vi "PID-testing.vi"() -> ()   [LabVIEW 2011]
uses:
  <vilib>/addons/control/pid/pid.llb/PID (DBL).vi
  <vilib>/Analysis/coordinate.llb/2D Cartesian Coordinate Rotation (Scalar).vi
  <vilib>/Analysis/NI_AALPro.lvlib
  <vilib>/addons/control/pid/NI_PID_pid.lvlib
panel:
  out "Y speed":dbl
  out "X speed":dbl
  in  "Y rate":dbl
  in  "X rate":dbl
  in  "stop":bool
  in  "Y 3":dbl
  in  "X 3":dbl
  in  "Y 2":dbl
  in  "X 2":dbl
  in  "Speed":dbl
  in  "Ramp":dbl
  in  "Y":dbl
  in  "X":dbl
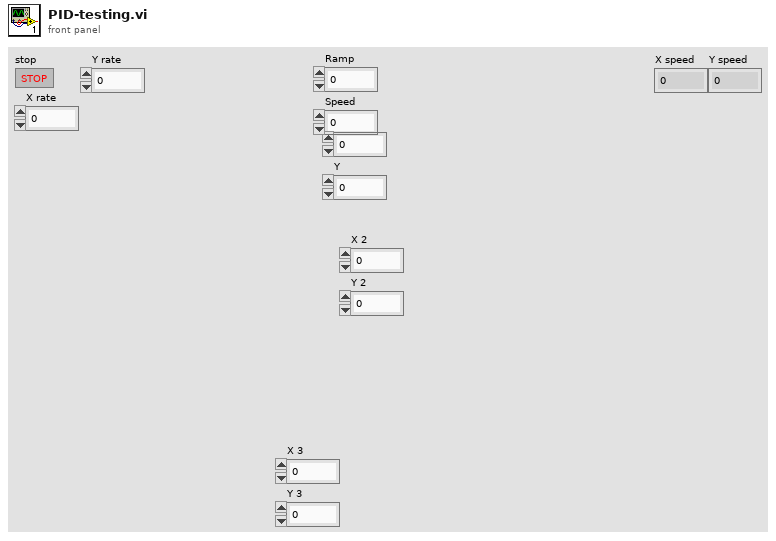
[diagram p1: front panel]
types:
  T1 = cluster{"proportional gain (Kc)":dbl, "integral time (Ti, min)":dbl, "derivative time (Td, min)":dbl}
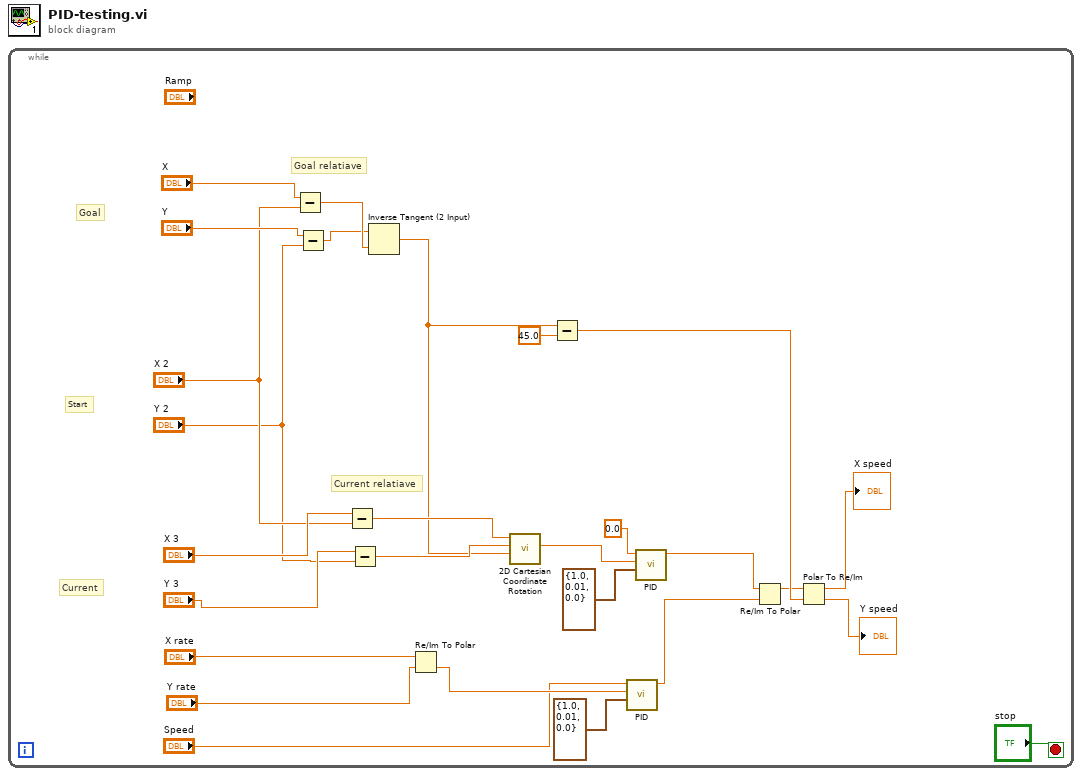
[diagram p0: block diagram]
diagram:
  n1 = while {
    stop <- "stop" stop-if-true
    # "Current relatiave"
    # "Goal relatiave"
    # "Current"
    # "Start"
    # "Goal"
    n2 = Subtract(x="X", y="X 2") -> (x-y=w21:dbl)
    n3 = Subtract(x="Y", y="Y 2") -> (x-y=w20:dbl)
    n4 = Subtract(x="X 3", y="X 2") -> (x-y=w19:dbl)
    n5 = Subtract(x="Y 3", y="Y 2") -> (x-y=w18:dbl)
    n6 = Inverse Tangent (2 Input)(1:w21, 2:w20) -> (0:w12:dbl)
    n7 = Re/Im To Polar(2:"Y rate", 3:"X rate") -> (0:w4:dbl)  [unwired: 1 out]
    n8 = call-poly <vilib>:"2D Cartesian Coordinate Rotation.vi"("theta"=w12, "y"=w18, "x"=w19) -> ("y out"=w8:dbl)  [unwired: 6 in, 2 out]
    n9 = Subtract(x=w12, y=45.0) -> (x-y=w13:dbl)
    n10 = call-poly <vilib>:"PID.vi"("PID gains"=T1 {"proportional gain (Kc)"=1.0, "integral time (Ti, min)"=0.01, "derivative time (Td, min)"=0.0}, "process variable"=w4, "setpoint"="Speed") -> ("output"=w5:dbl)  [unwired: 7 in, 1 out]
    n11 = call-poly <vilib>:"PID.vi"("PID gains"=T1 {"proportional gain (Kc)"=1.0, "integral time (Ti, min)"=0.01, "derivative time (Td, min)"=0.0}, "process variable"=w8, "setpoint"=0.0) -> ("output"=w9:dbl)  [unwired: 7 in, 1 out]
    n12 = Re/Im To Polar(2:w5, 3:w9) -> (1:w11:dbl)  [unwired: 1 out]
    n13 = Polar To Re/Im(2:w13, 3:w11) -> (0:→"Y speed":dbl, 1:→"X speed":dbl)
  }
